vi "Joystick_Debugger2.vi"() -> ()   [LabVIEW 2011]
doc: "This VI show how to use the basic functions in the Input Device palette. It will show information about all the joysticks, keyboards and mice attached to the system (number of axes, buttons, pov, and the name). It will also give the current information for the first joystick attached to the system (location and button pressed). The current information for the first keyboard and mouse will also be displayed."
uses:
  <vilib>/Utility/inputDevices.llb/closeJoystick.vi
  <vilib>/Utility/inputDevices.llb/closeKeyboard.vi
  <vilib>/Utility/inputDevices.llb/closeMouse.vi
  <vilib>/Utility/inputDevices.llb/joystickAcquire.vi
  <vilib>/Utility/inputDevices.llb/keyboardAcquire.vi
  <vilib>/Utility/inputDevices.llb/mouseAcquire.vi
panel:
  out "Button 12":bool
  out "Button 11":bool
  out "Button 10":bool
  out "Button 9":bool
  out "Button 8":bool
  out "Button 7":bool
  out "Button 6":bool
  out "Button 5":bool
  out "Button 4":bool
  out "Button 3":bool
  out "Button 2":bool
  out "V-Axis":i32
  out "Y-Rot":i32
  out "Z-Rot":i32
  out "U-Axis":i32
  out "X-Rot":i32
  out "Z-axis":i32
  in  "Message":string="LabVIEW was unable\nto detect a joystick."
  in  "Button":string="Continue"
  out "Left Button Pressed":bool
  out "Axis Info":T1
  out "Mouse Info":T2(array[cluster])
  out "Keys Pressed":T3(array[ring])
  out "Key Info":T4(array[cluster])
  out "X-axis":i32(slide) scale=-33000.0..33000.0
  out "Y-axis":i32(slide) scale=-33000.0..33000.0
  out "Joystick Info":T5(array[cluster])
  out "POV 1":i32
  out "Button 1":bool
  in  "stop":bool
  # "JOYSTICKS"
  # "KEYBOARD/KEYPADS"
  # "MICE"
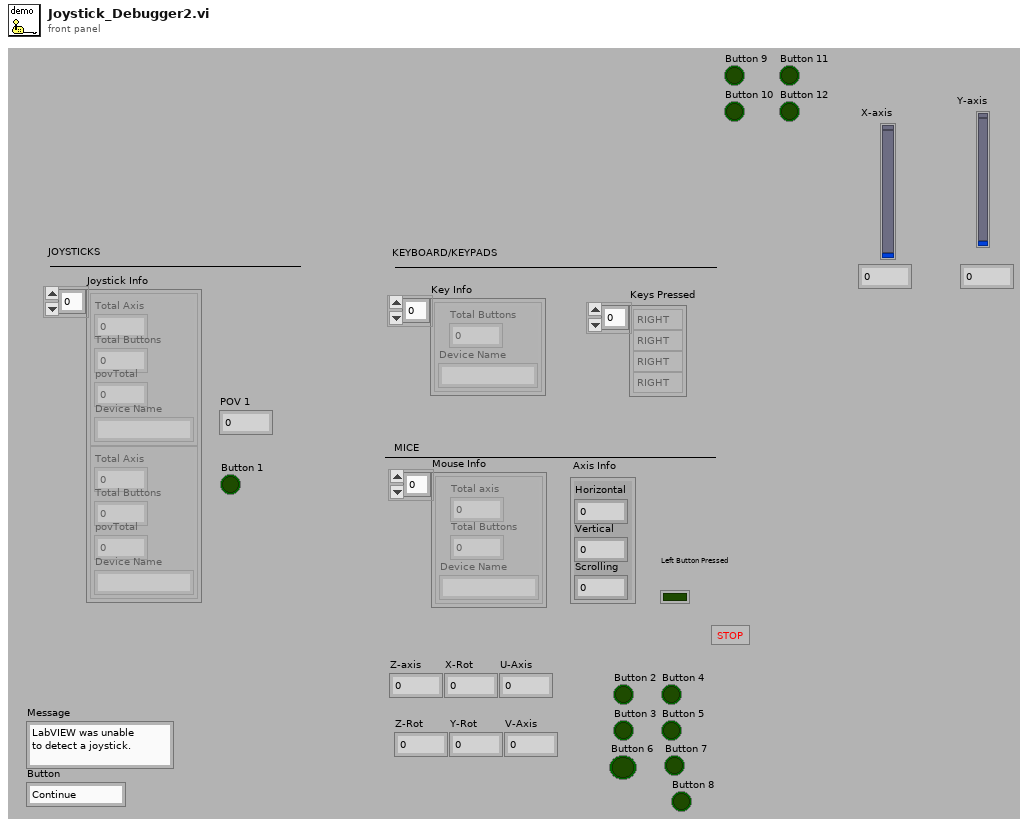
[diagram p1: front panel]
types:
  T1 = cluster{"Horizontal":i32, "Vertical":i32, "Scrolling":i32}
  T2 = cluster{"Total axis":u32, "Total Buttons":u32, "Device Name":string}[]
  T3 = enum16{"0", "1", "2", "3", "4", "5", "6", "7", "8", "9", "A", "B", "C", "D", "E", "F", "G", "H", "I", "J", "K", "L", "M", "N", "O", "P", "Q", "R", "S", "T", "U", "V", "W", "X", "Y", "Z", "F1", "F2", "F3", "F4", "F5", "F6", "F7", "F8", "F9", "F10", "F11", "F12", "F13", "F14", "F15", "ADD", "BACK", "BACKSLASH", "CAPITAL", "COMMA", "DECIMAL", "DELETE", "DIVIDE", "DOWN", "END", "EQUALS", "ESCAPE", "GRAVE (`)", "HOME", "INSERT", "LBRACKET", "LCONTROL", "LEFT", "L ALT", "LSHIFT", "LWIN", "MINUS", "MULTIPLY", "NEXT", "NUMLOCK", "NUMPAD_0", "NUMPAD_1", "NUMPAD_2", "NUMPAD_3", "NUMPAD_4", "NUMPAD_5", "NUMPAD_6", "NUMPAD_7", "NUMPAD_8", "NUMPAD_9", "PAUSE", "PERIOD", "PRIOR (PG UP)", "RBRACKET", "RCONTROL", "RETURN", "RIGHT", "R ALT", "RSHIFT", "RWIN", "SCROLL", "SEMICOLON", "SLASH", "SPACE", "SUBTRACT", "TAB", "UP", "ENTER (num pad)", "' (quote)"}[]
  T4 = cluster{"Total Buttons":u32, "Device Name":string}[]
  T5 = cluster{"Total Axis":u32, "Total Buttons":u32, "povTotal":u32, "Device Name":string}[]
  T6 = cluster{"axes total":u32, "buttons total":u32, "device name":string}[]
  T7 = cluster{"buttons total":u32, "device name":string}[]
  T8 = cluster{"axes total":u32, "buttons total":u32, "pov total":u32, "device name":string}[]
  T9 = cluster{"X axis":i32, "Y axis":i32, "Z axis":i32, "X axis rotation":i32, "Y axis rotation":i32, "Z axis rotation":i32, "U axis":i32, "V axis":i32}
  T10 = cluster{"button 1":bool, "button 2":bool, "button 3":bool, "button 4":bool, "button 5":bool, "button 6":bool, "button 7":bool, "button 8":bool, "button 9":bool, "button 10":bool, "button 11":bool, "button 12":bool, "button 13":bool, "button 14":bool, "button 15":bool, "button 16":bool, "button 17":bool, "button 18":bool, "button 19":bool, "button 20":bool, "button 21":bool, "button 22":bool, "button 23":bool, "button 24":bool, "button 25":bool, "button 26":bool, "button 27":bool, "button 28":bool, "button 29":bool, "button 30":bool, "button 31":bool, "button 32":bool}
  T11 = cluster{"pov 1":i32, "pov 2":i32, "pov 3":i32, "pov 4":i32}
  T12 = cluster{"button 1":bool, "button 2":bool, "button 3":bool, "button 4":bool}
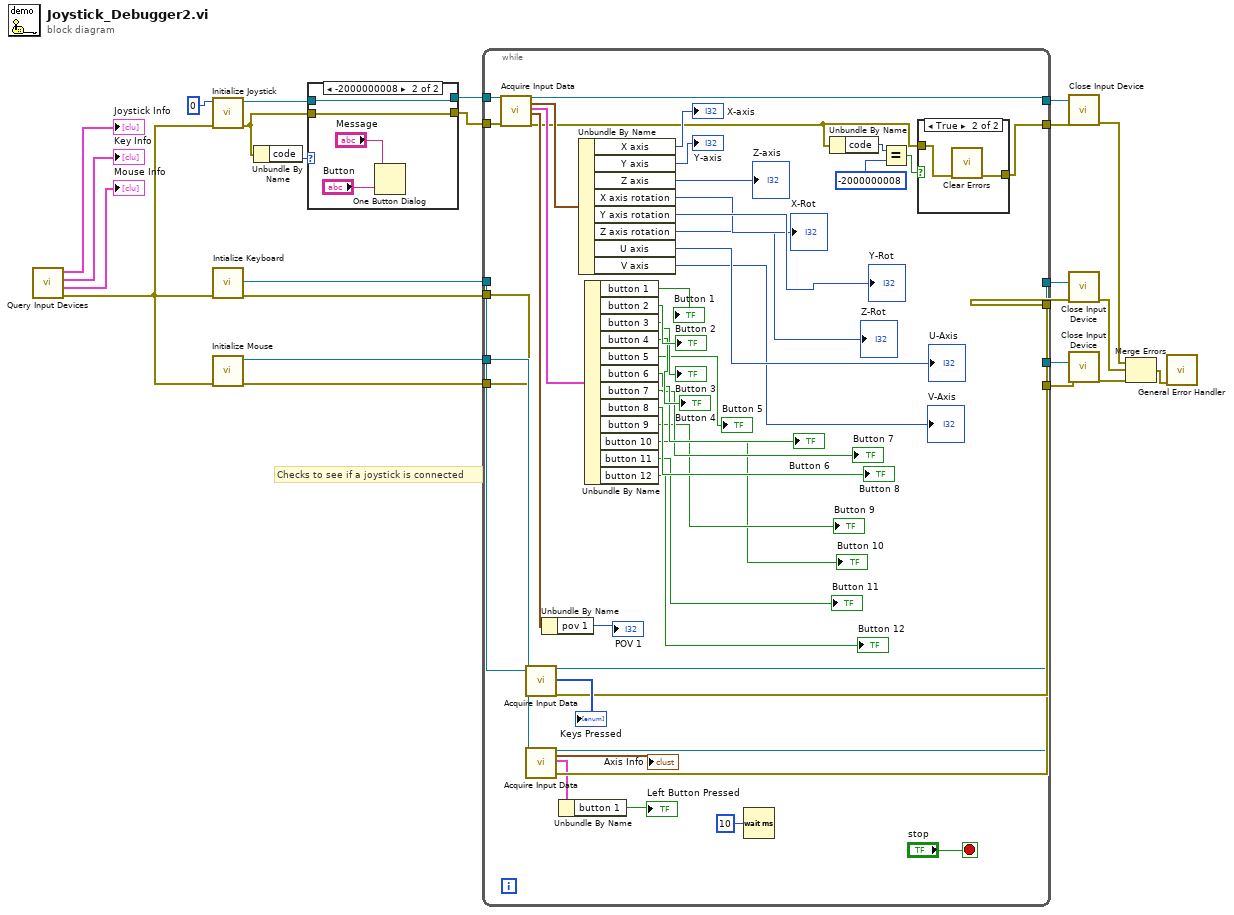
[diagram p0: block diagram]
diagram:
  # "Checks to see if a joystick is connected"
  n1 = call <vilib>:"Query Input Devices.vi"() -> ("error out"=w20:errorcluster, "mouse info"=→"Mouse Info":T6, "key info"=→"Key Info":T7, "joystick info"=→"Joystick Info":T8)  [unwired: 1 in, 7 out]
  n2 = call <vilib>:"Initialize Joystick.vi"("error in (no error)"=w20, "device index"=0) -> ("error out"=w3:errorcluster, "device ID"=w4:refnum<k1>)  [unwired: 8 out]
  n3 = call <vilib>:"Intialize Keyboard.vi"("error in (no error)"=w20) -> ("error out"=w22:errorcluster, "device ID"=w24:refnum<k1>)  [unwired: 9 out]
  n4 = call <vilib>:"Initialize Mouse.vi"("error in (no error)"=w20) -> ("error out"=w21:errorcluster, "device ID"=w23:refnum<k1>)  [unwired: 9 out]
  n5 = Unbundle By Name(w3) -> ("code"=w5:i32)
  n6 = case shown="-2000000008" w5 {
    tunnel: w3 -> [w26 w28]
    tunnel: [w26 w28] -> w2
    tunnel: w4 -> [w25 w27]
    tunnel: [w25 w27] -> w1
    frame 0, Default {
    }
    frame -2000000008 {
      n7 = One Button Dialog(message="Message", button name ("OK")="Button") -> ()  [unwired: 1 out]
    }
  }
  n8 = while {
    tunnel: [w64] -> w10
    tunnel: [w57] -> w11
    tunnel: [w65] -> w12
    tunnel: [w51] -> w14
    tunnel: w21 -> [w66]
    tunnel: w22 -> [w67]
    tunnel: w23 -> [w68]
    tunnel: [w59] -> w15
    tunnel: [w58] -> w13
    tunnel: w24 -> [w56]
    tunnel: w2 -> [w49]
    tunnel: w1 -> [w48]
    stop <- "stop" stop-if-true
    n9 = call-poly <vilib>:"Acquire Input Data.vi"("device ID"=w48, "error in (no error)"=w49) -> ("device ID"=w59:refnum<k1>, "axis info"=w76:T9, "button info"=w73:T10, "direction info"=w71:T11, "error out"=w50:errorcluster)  [unwired: 13 out]
    n10 = call-poly <vilib>:"Acquire Input Data.vi"("device ID"=w56, "error in (no error)"=w67) -> ("device ID"=w58:refnum<k1>, "keys pressed"=→"Keys Pressed":T3, "error out"=w65:errorcluster)  [unwired: 15 out]
    n11 = call-poly <vilib>:"Acquire Input Data.vi"("device ID"=w68, "error in (no error)"=w66) -> ("device ID"=w57:refnum<k1>, "axis info"=→"Axis Info":T1, "button info"=w63:T12, "error out"=w64:errorcluster)  [unwired: 1 in, 13 out]
    n12 = Unbundle By Name(w71) -> ("pov 1"=→"POV 1":i32)
    n13 = Unbundle By Name(w63) -> ("button 1"=→"Left Button Pressed":bool)
    n14 = Unbundle By Name(w76) -> ("X axis"=→"X-axis":i32, "Y axis"=→"Y-axis":i32, "Z axis"=→"Z-axis":i32, "X axis rotation"=→"X-Rot":i32, "Y axis rotation"=→"Y-Rot":i32, "Z axis rotation"=→"Z-Rot":i32, "U axis"=→"U-Axis":i32, "V axis"=→"V-Axis":i32)
    n15 = Unbundle By Name(w73) -> ("button 1"=→"Button 1":bool, "button 2"=→"Button 2":bool, "button 3"=→"Button 3":bool, "button 4"=→"Button 4":bool, "button 5"=→"Button 5":bool, "button 6"=→"Button 6":bool, "button 7"=→"Button 7":bool, "button 8"=→"Button 8":bool, "button 9"=→"Button 9":bool, "button 10"=→"Button 10":bool, "button 11"=→"Button 11":bool, "button 12"=→"Button 12":bool)
    n16 = Wait (ms)(milliseconds to wait=u32 10) -> ()  [unwired: 1 out]
    n17 = Unbundle By Name(w50) -> ("code"=w54:i32)
    n18 = Equal?(x=w54, y=-2000000008) -> (x = y?=w52:bool)
    n19 = case shown="True" w52 {
      tunnel: w50 -> [w77 w79]
      tunnel: [w77 w78] -> w51
      frame False {
      }
      frame True {
        n20 = call <vilib>:"Clear Errors.vi"("error in (no error)"=w79) -> ("error out"=w78:errorcluster)  [unwired: 6 out]
      }
    }
  }
  n21 = call-poly <vilib>:"Close Input Device.vi"("error in (no error)"=w14, "device ID"=w15) -> ("error out"=w6:errorcluster)  [unwired: 8 out]
  n22 = call-poly <vilib>:"Close Input Device.vi"("error in (no error)"=w12, "device ID"=w13) -> ("error out"=w7:errorcluster)  [unwired: 8 out]
  n23 = call-poly <vilib>:"Close Input Device.vi"("error in (no error)"=w10, "device ID"=w11) -> ("error out"=w9:errorcluster)  [unwired: 8 out]
  n24 = Merge Errors(w6, w7, w9) -> (w16:errorcluster)
  n25 = call <vilib>:"General Error Handler.vi"("error in (no error)"=w16) -> ()  [unwired: 1 in, 14 out]
